vi "GenCM-Read config.vi"(0 "AO Map":T1, 1 "min slot":u32=2, 5 "AI Map":T1, 7 "config name":string="Connections", 9 "slot ctl refs":refnum<vi>[](array[refnum]), 11 "error in (no error)":errorcluster, 12 "Outputs":string[](array[string]), 13 "Inputs":string[](array[string])) -> (4 "Hide unused?":bool, 15 "error out":errorcluster)   [LabVIEW 2015]
uses:
  Type Defs/General PXISlot XControl/PXISlotGP.xctl
  PXI DAQ VIs/Utility VIs/Array Dimensions (2D).vi
  <vilib>/Utility/config.llb/Read Key (I32).vi
  <vilib>/Utility/config.llb/Read Key (Boolean).vi
  <vilib>/Utility/config.llb/NI_LVConfig.lvlib
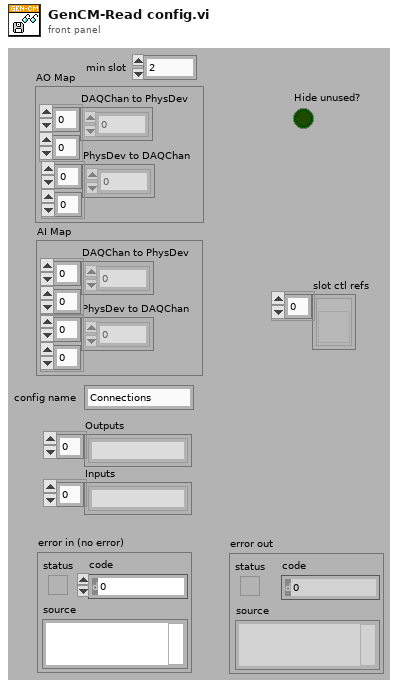
[diagram p1: front panel]
types:
  T1 = cluster{"DAQChan to PhysDev":i32[][], "PhysDev to DAQChan":i32[][]}
  T2 = typedef "NI_LVConfig.lvlib/Config Data RefNum.ctl" = refnum<k1>
  T3 = cluster{"DAQChan to PhysDev":i32[][], "PhysDev to DAQChan":i32[][]}[]
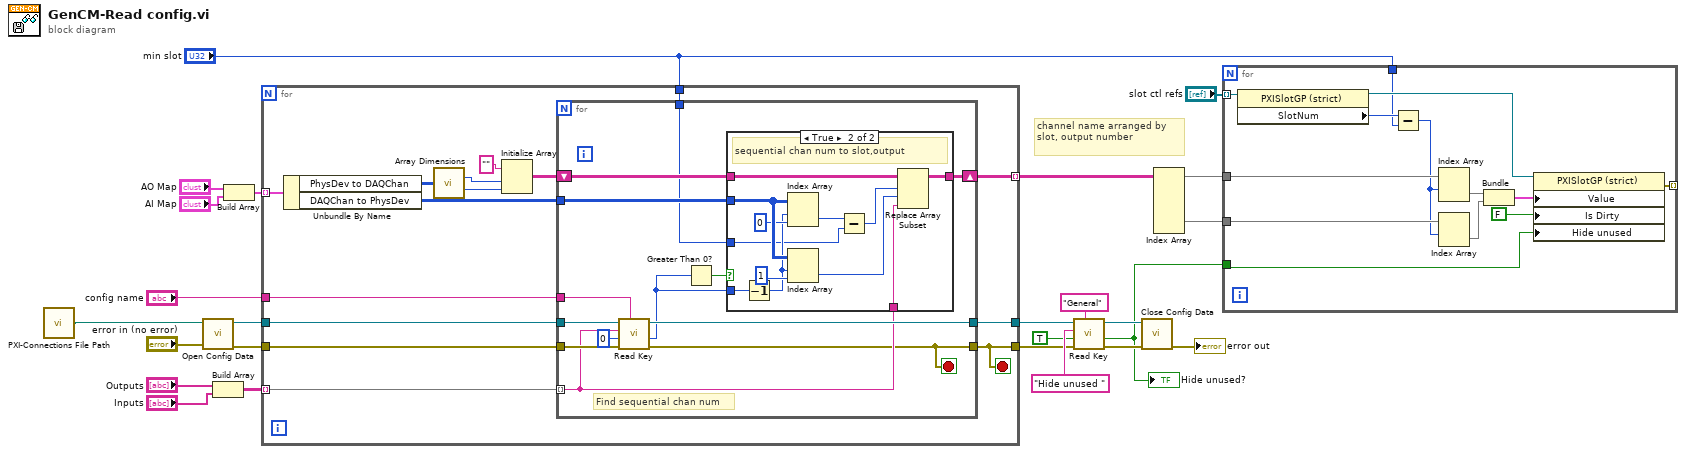
[diagram p0: block diagram]
diagram:
  # "channel name arranged by slot, output number"
  n1 = call "PXI-Connections File Path.vi"() -> ("Path"=w2:path)  [unwired: 1 in]
  n2 = call <vilib>:"Open Config Data.vi"("error in (no error)"="error in (no error)", "configuration file path"=w2) -> ("error out"=w6:errorcluster, "refnum"=w24:T2)  [unwired: 7 in, 1 out]
  n3 = Build Array("Outputs", "Inputs") -> (w4:string[][])
  n4 = Build Array("AO Map", "AI Map") -> (w13:T3)
  n5 = for {
    tunnel: w4 -> [w28] mode=indexing
    tunnel: w6 -> [w40]
    tunnel: w24 -> [w39]
    tunnel: w13 -> [w38] mode=indexing
    tunnel: [w32] -> w21 mode=indexing
    tunnel: "config name" -> [w31]
    tunnel: [w29] -> w8
    tunnel: [w27] -> w7
    tunnel: "min slot" -> [w26]
    stop <- w27 stop-if-true
    n6 = Unbundle By Name(w38) -> ("PhysDev to DAQChan"=w36:i32[][], "DAQChan to PhysDev"=w37:i32[][])
    n7 = call-poly "Array Dimensions.vi"("2D Array"=w36) -> ("# rows"=w35:i32, "# columns"=w34:i32)  [unwired: 13 in]
    n8 = Initialize Array("", w35, w34) -> (w33:string[][])
    n9 = for {
      tunnel: w28 -> [w43] mode=indexing
      tunnel: w39 -> [w52]
      tunnel: w31 -> [w51]
      tunnel: w37 -> [w49]
      shift-right: [w47] -> w32
      shift-left: w33 -> [w48]
      tunnel: [w46] -> w29
      tunnel: w40 -> [w53]
      tunnel: [w42] -> w27
      tunnel: w26 -> [w41]
      stop <- w42 stop-if-true
      # "Find sequential chan num"
      n10 = call-poly <vilib>:"Read Key.vi"("section"=w51, "error in (no error)"=w53, "default value"=0, "key"=w43, "refnum"=w52) -> ("error out"=w42:errorcluster, "value"=w44:i32, "refnum out"=w46:T2)  [unwired: 3 in, 1 out]
      n11 = Greater Than 0?(x=w44) -> (x > 0?=w45:bool)
      n12 = case shown="True" w45 {
        tunnel: w49 -> [_ w66]
        tunnel: w48 -> [w54 w65]
        tunnel: [w54 w64] -> w47
        tunnel: w44 -> [_ w58]
        tunnel: w43 -> [_ w56]
        tunnel: w41 -> [_ w55]
        frame False {
        }
        frame True {
          # "sequential chan num to slot,output"
          n13 = Decrement(x=w58) -> (x-1=w57:i32)
          n14 = Index Array(array=w66, index (row)=w57, index (col)=0 ("length")) -> (element=w59:i32)
          n15 = Index Array(array=w66, index (row)=w57, index (col)=1 ("length")) -> (element=w61:i32)
          n16 = Subtract(x=w59, y=w55) -> (x-y=w60:u32)
          n17 = Replace Array Subset(array=w65, new element=w56, index (row)=w60, index (col)=w61) -> (w64:string[][])
        }
      }
    }
  }
  n18 = call-poly <vilib>:"Read Key.vi"("section"="General", "error in (no error)"=w7, "default value"=TRUE, "key"="Hide unused ", "refnum"=w8) -> ("error out"=w20:errorcluster, "value"=w15:bool, "refnum out"=w19:T2)  [unwired: 3 in, 1 out]
  "Hide unused?" <- w15
  n19 = call <vilib>:"Close Config Data.vi"("error in (no error)"=w20, "refnum"=w19) -> ("error out"=→"error out":errorcluster)  [unwired: 8 in, 1 out]
  n20 = Index Array(array=w21) -> (element #1=w10:string[][], element #2=w9:string[][])  [unwired: 6 in]
  n21 = for {
    tunnel: "slot ctl refs" -> [w78] mode=indexing
    tunnel: w10 -> [w73]
    tunnel: w9 -> [w76]
    tunnel: w15 -> [w69]
    tunnel: "min slot" -> [w68]
    tunnel: [w67] -> _ mode=indexing
    n22 = property class="PXISlotGP (strict)"(reference=w78) -> (reference out=w77:refnum<vi>, "SlotNum"=w75:i32)  [unwired: 1 in, 1 out]
    n23 = Subtract(x=w75, y=w68) -> (x-y=w72:u32)
    n24 = Index Array(array=w73, index (row)=w72) -> (element=w71:string[])  [unwired: 1 in]
    n25 = Index Array(array=w76, index (row)=w72) -> (element=w74:string[])  [unwired: 1 in]
    n26 = Bundle(w71, w74) -> (w79:cluster{string[], string[]})  [unwired: 1 in]
    n27 = property class="PXISlotGP (strict)"(reference=w77, "Value"=w79, "Is Dirty"=FALSE, "Hide unused"=w69) -> (error out=w67:errorcluster)  [unwired: 1 in, 1 out]
  }
